vi "Decimal to SNAFU.vi"(11 "Decimal":i64) -> (3 "SNAFU":string)   [LabVIEW 2021, in "d25.lvlib"]
uses:
  d25.lvlib
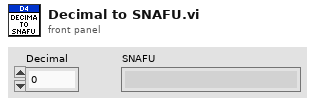
[diagram p1: front panel]
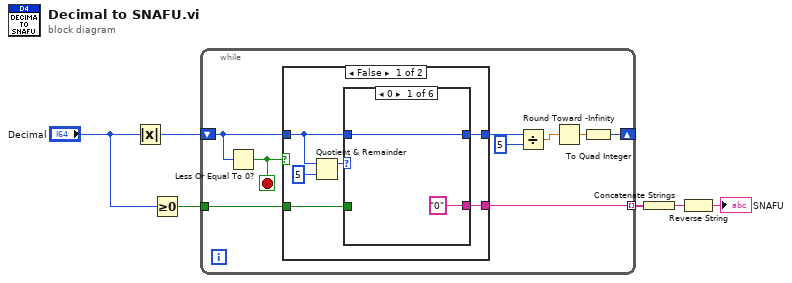
[diagram p0: block diagram]
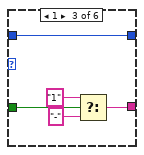
[diagram p3: hidden frame]
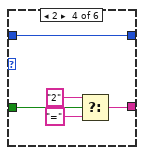
[diagram p4: hidden frame]
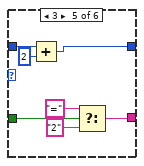
[diagram p5: hidden frame]
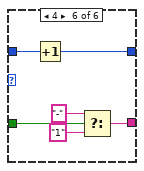
[diagram p6: hidden frame]
diagram:
  n1 = Absolute Value(x="Decimal") -> (abs(x)=w3:i64)
  n2 = Greater Or Equal To 0?(x="Decimal") -> (x >= 0?=w1:bool)
  n3 = while {
    shift-right: [w8] -> _
    shift-left: w3 -> [w14]
    tunnel: [w13] -> w5 mode=indexing
    tunnel: w1 -> [w7]
    stop <- w12 stop-if-true
    n4 = Less Or Equal To 0?(x=w14) -> (x <= 0?=w12:bool)
    n5 = case shown="False" w12 {
      tunnel: [w21 _] -> w13
      tunnel: [w17 w48] -> w15
      tunnel: w14 -> [w18 w48]
      tunnel: w7 -> [w16 _]
      frame False {
        n6 = Quotient & Remainder(x=w18, y=i64 5) -> (x-y*floor(x/y)=w19:i64)  [unwired: 1 out]
        n7 = case shown="0" w19 {
          tunnel: ["0" _ w27 w33 w38 w45] -> w21
          tunnel: w18 -> [w22 w24 w28 w34 w41 w47]
          tunnel: [w22 w24 w28 w34 w40 w46] -> w17
          tunnel: w16 -> [_ _ w26 w31 w36 w43]
          frame 0 {
          }
          frame Default {
          }
          frame 1 {
            n8 = Select(t="1", s=w26, f="-") -> (s? t:f=w27:string)
          }
          frame 2 {
            n9 = Select(t="2", s=w31, f="=") -> (s? t:f=w33:string)
          }
          frame 3 {
            n10 = Add(x=w41, y=i64 2) -> (x+y=w40:i64)
            n11 = Select(t="=", s=w36, f="2") -> (s? t:f=w38:string)
          }
          frame 4 {
            n12 = Increment(x=w47) -> (x+1=w46:i64)
            n13 = Select(t="-", s=w43, f="1") -> (s? t:f=w45:string)
          }
        }
      }
      frame True {
      }
    }
    n14 = Divide(x=w15, y=i64 5) -> (x/y=w11:dbl)
    n15 = Round Toward -Infinity(1:w11) -> (0:w9:dbl)
    n16 = To Quad Integer(1:w9) -> (0:w8:i64)
  }
  n17 = Concatenate Strings(w5) -> (w6:string)
  n18 = Reverse String(1:w6) -> (0:→"SNAFU":string)
